vi "ReadFileType.vi"(8 "error in (no error)":errorcluster, 11 "object in":refnum<class "DataType.lvclass">) -> (0 "error out":errorcluster, 2 "File Type":T1, 3 "object out":refnum<class "DataType.lvclass">)   [LabVIEW 2024, in "DataType.lvclass"]
uses:
  <resource>/Framework/Providers/Open_GDS/ClassProviders/Provider_LvNativeClass/Templates/NativeBaseTemplate/NativeBaseTemplate.lvclass/NativeBaseTemplate.ctl
  DataType.lvclass
  DataType.lvclass/DataType.ctl
  Support/Type Def/File Type.ctl
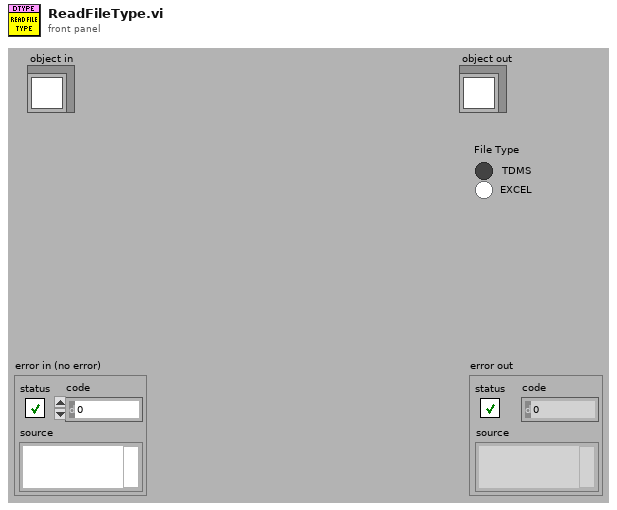
[diagram p1: front panel]
types:
  T1 = typedef "File Type.ctl" = enum32{"TDMS", "EXCEL"}
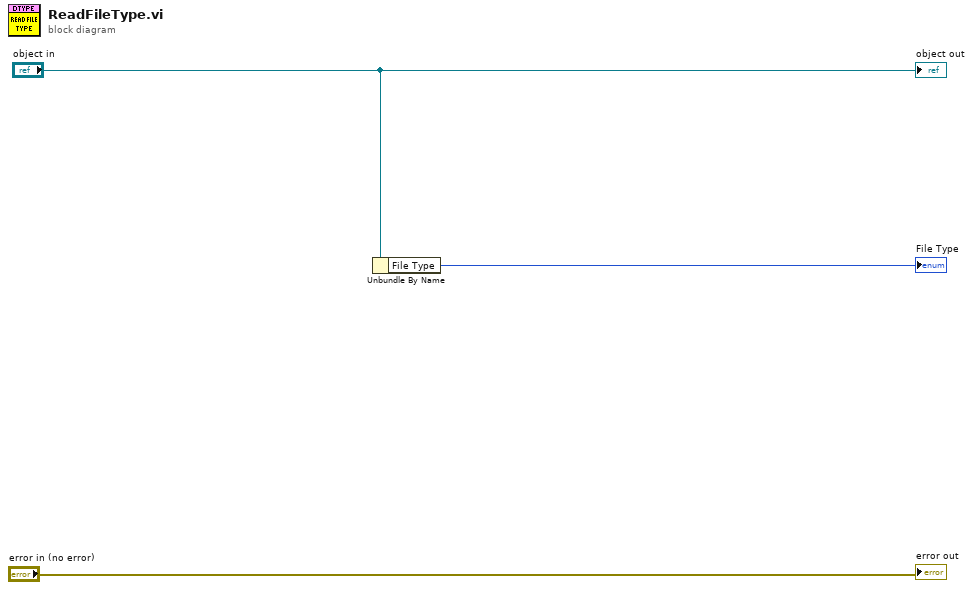
[diagram p0: block diagram]
diagram:
  n1 = Unbundle By Name("object in") -> ("File Type"=→"File Type":T1)
  "error out" <- "error in (no error)"
  "object out" <- "object in"
